vi "ParameterInfo.vi"(0 "Data name":string) -> (1 "Array level":i32, 2 "Interceptor style":string)   [LabVIEW 2013]
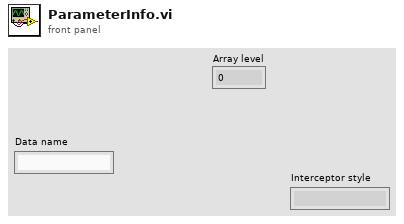
[diagram p1: front panel]
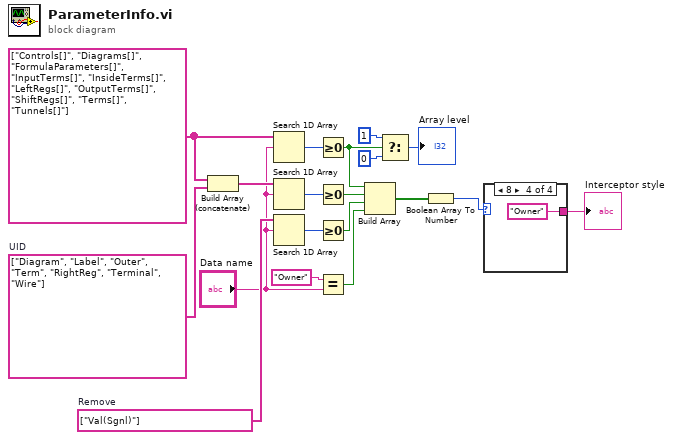
[diagram p0: block diagram]
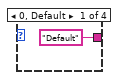
[diagram p2: hidden frame]
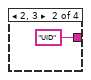
[diagram p3: hidden frame]
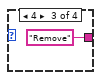
[diagram p4: hidden frame]
diagram:
  w8 = string[] ["Val(Sgnl)"]  # Remove
  w5 = string[] ["Diagram", "Label", "Outer", "Term", "RightReg", "Terminal", "Wire"]  # UID
  w6 = string[] ["Controls[]", "Diagrams[]", "FormulaParameters[]", "InputTerms[]", "InsideTerms[]", "LeftRegs[]", "OutputTerms[]", "ShiftRegs[]", "Terms[]", "Tunnels[]"]
  n1 = Build Array (concatenate)(w6, w5) -> (w4:string[])
  n2 = Search 1D Array(1D array=w6, element="Data name") -> (index of element=w19:i32)  [unwired: 1 in]
  n3 = Search 1D Array(1D array=w4, element="Data name") -> (index of element=w15:i32)  [unwired: 1 in]
  n4 = Search 1D Array(1D array=w8, element="Data name") -> (index of element=w9:i32)  [unwired: 1 in]
  n5 = Greater Or Equal To 0?(x=w19) -> (x >= 0?=w14:bool)
  n6 = Greater Or Equal To 0?(x=w15) -> (x >= 0?=w13:bool)
  n7 = Greater Or Equal To 0?(x=w9) -> (x >= 0?=w7:bool)
  n8 = Equal?(x="Owner" ("Remove"), y="Data name") -> (x = y?=w1:bool)
  n9 = Build Array(w14, w13, w7, w1) -> (w12:bool[])
  n10 = Select(t=1, s=w14, f=0) -> (s? t:f=→"Array level":i32)
  n11 = Boolean Array To Number(Boolean array=w12) -> (number=w11:u32)
  n12 = case shown="8" w11 {
    tunnel: ["Default" "UID" "Remove" "Owner"] -> w10
    frame 0, Default {
    }
    frame 2, 3 {
    }
    frame 4 {
    }
    frame 8 {
    }
  }
  "Interceptor style" <- w10
